vi "DSF.Execution.Runtime.Plugin Manager.Query Disk.Classes.Plugin.vi"(8 "error in (no error)":errorcluster, 10 "Plugin name":string, 11 "Plugin Manager in":refnum<class "DSF.Engine.Runtime.Plugin Manager.lvclass">) -> (0 "error out":errorcluster, 2 "Plugin class paths":path[](array[path]), 3 "Plugin Manager out":refnum<class "DSF.Engine.Runtime.Plugin Manager.lvclass">)   [LabVIEW 2016, in "DSF.Engine.lvlib" / "DSF.Engine.Runtime.Plugin Manager.lvclass"]
uses:
  DSF.Engine.Runtime.Plugin Manager.lvclass
  DSF.Engine.Runtime.Plugin Manager.lvclass/DSF.Engine.Runtime.Plugin Manager.ctl
  DSF.Execution.Runtime.Plugin Manager.Get Plugins Folder.vi
  <vilib>/Utility/libraryn.llb/Recursive File List.vi
  <vilib>/Utility/libraryn.llb/Check if File or Folder Exists.vi
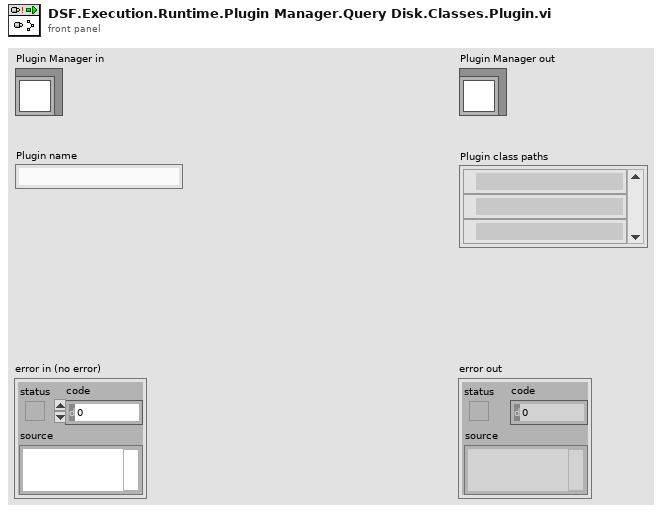
[diagram p1: front panel]
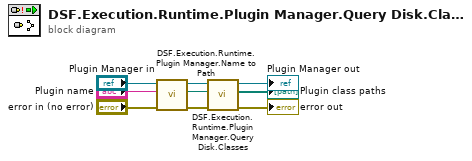
[diagram p0: block diagram]
diagram:
  n1 = call "DSF.Execution.Runtime.Plugin Manager.Name to Path.vi"("error in (no error)"="error in (no error)", "Plugin name"="Plugin name", "Plugin Manager in"="Plugin Manager in") -> ("error out"=w6:errorcluster, "Plugin folder"=w4:path, "Plugin Manager out"=w5:refnum<class "DSF.Engine.Runtime.Plugin Manager.lvclass">)  [unwired: 6 in]
  n2 = call "DSF.Execution.Runtime.Plugin Manager.Query Disk.Classes.vi"("error in (no error)"=w6, "folder"=w4, "Plugin Manager in"=w5) -> ("error out"=→"error out":errorcluster, "class paths"=→"Plugin class paths":path[], "Plugin Manager out"=→"Plugin Manager out":refnum<class "DSF.Engine.Runtime.Plugin Manager.lvclass">)  [unwired: 6 in]
